vi "Launcher.vi"() -> ()   [LabVIEW 2024]
uses:
  SpeakTurkish/SpeakTurkish.lvclass
  LearnByVisual/LearnByVisual.lvclass
  LearnByReading/LearnByReading.lvclass
  SpeakEnglish/SpeakEnglish.lvclass
  <vilib>/Utility/miscctls.llb/LVRectTypeDef.ctl
  Person/Person.lvclass
panel:
  out "Profile Picture":picture
  in  "Stop":bool
  in  "Person":enum16{"JOHN", "MEHMET", "MARIE"}(ring)
  out "Learning Style":string
  out "Language":string
  out "Name":string
  # "NAME"
  # "SPEAKS"
  # "LEARNS BY"
  # "CHOOSE PERSON"
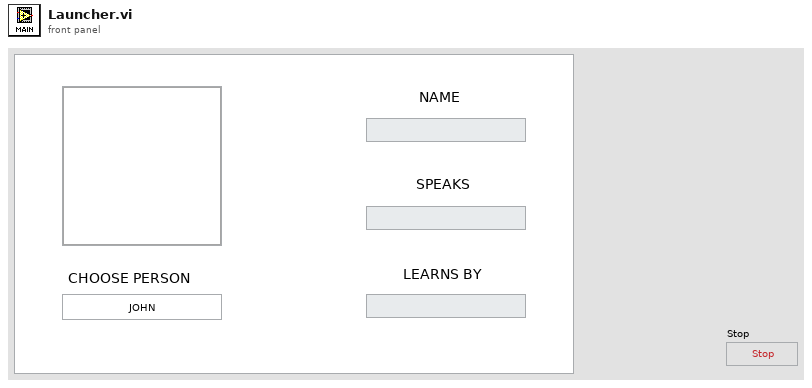
[diagram p1: front panel]
types:
  T1 = typedef "LVRectTypeDef.ctl" = cluster{"Left":i16, "Top":i16, "Right":i16, "Bottom":i16}
  T2 = typedef "LVBoundsTypeDef.ctl" = cluster{"Width":u32, "Height":u32}
  T3 = typedef "imagedata.ctl" = cluster{"image type":i32, "image depth":i32, "image":u8[], "mask":u8[], "colors":u32[], "Rectangle":cluster{"left":i16, "top":i16, "right":i16, "bottom":i16}}
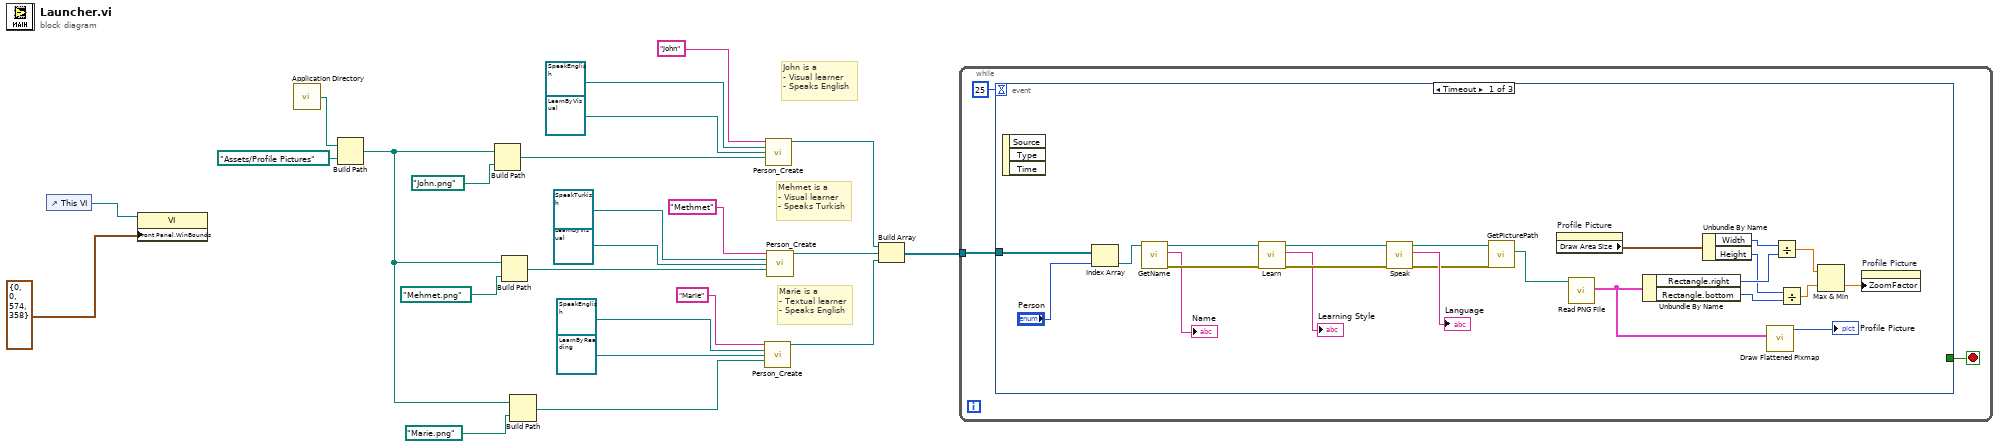
[diagram p0: block diagram]
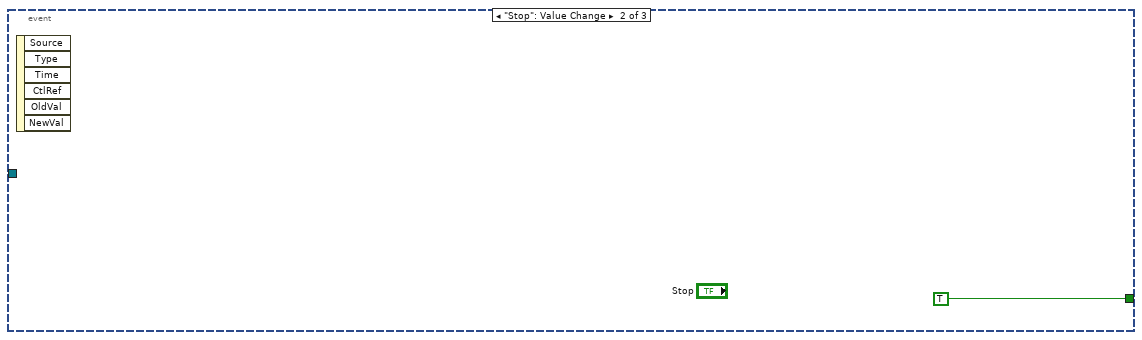
[diagram p2: hidden frame]
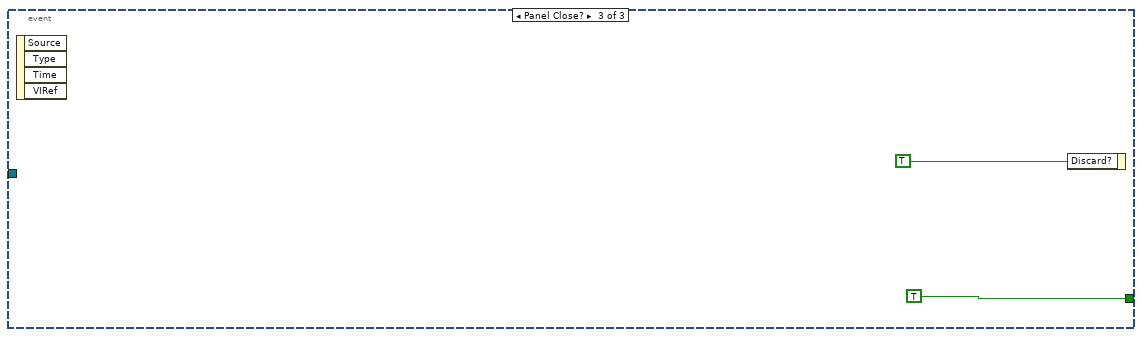
[diagram p3: hidden frame]
diagram:
  # "Marie is a\n- Textual learner\n- Speaks English"
  # "Mehmet is a\n- Visual learner\n- Speaks Turkish"
  # "John is a\n- Visual learner\n- Speaks English"
  n1 = control-ref of="This VI"() -> (w5:refnum<vi>)
  n2 = property class="VI"(reference=w5, "Front Panel.WinBounds"=T1 {"Left"=0, "Top"=0, "Right"=574, "Bottom"=358} ("Front Panel Window:Window Bounds")) -> ()  [unwired: 1 in, 2 out]
  n3 = call <vilib>:"Application Directory.vi"() -> ("Application Directory"=w2:path)
  n4 = Build Path(base path=w2, name or relative path=path "Assets/Profile Pictures") -> (appended path=w3:path)
  n5 = Build Path(base path=w3, name or relative path=path "John.png") -> (appended path=w17:path)
  n6 = Build Path(base path=w3, name or relative path=path "Mehmet.png") -> (appended path=w11:path)
  n7 = Build Path(base path=w3, name or relative path=path "Marie.png") -> (appended path=w6:path)
  n8 = call "Person_Create.vi"("Name"="Marie", "ISpeakBehaviour"=refnum<class "SpeakEnglish.lvclass"> refnum ("SpeakEnglish"), "ILearnBehaviour"=refnum<class "LearnByReading.lvclass"> refnum ("LearnByReading"), "PicturePath"=w6) -> ("reference out"=w22:refnum<class "Person.lvclass">)  [unwired: 10 in, 1 out]
  n9 = call "Person_Create.vi"("Name"="John", "ISpeakBehaviour"=refnum<class "SpeakEnglish.lvclass"> refnum ("SpeakEnglish"), "ILearnBehaviour"=refnum<class "LearnByVisual.lvclass"> refnum ("LearnByVisual"), "PicturePath"=w17) -> ("reference out"=w24:refnum<class "Person.lvclass">)  [unwired: 10 in, 1 out]
  n10 = call "Person_Create.vi"("Name"="Methmet", "ISpeakBehaviour"=refnum<class "SpeakTurkish.lvclass"> refnum ("SpeakTurkish"), "ILearnBehaviour"=refnum<class "LearnByVisual.lvclass"> refnum ("LearnByVisual"), "PicturePath"=w11) -> ("reference out"=w23:refnum<class "Person.lvclass">)  [unwired: 10 in, 1 out]
  n11 = Build Array(w24, w23, w22) -> (w21:refnum<class "Person.lvclass">[])
  n12 = while {
    tunnel: w21 -> [w26]
    stop <- w27 stop-if-true
    n13 = event shown="[0] Timeout" {
      selector: _ -> [_ _ _]
      dyn-events: _ -> [_ _ _]
      timeout: 25 -> [_ _ _]
      tunnel: [_ TRUE TRUE] -> w27
      tunnel: w26 -> [w50 _ _]
      event Timeout {
        n14 = event-data() -> ()  [unwired: 1 in, 3 out]
        n15 = Index Array(array=w50, index="Person") -> (element=w44:refnum<class "Person.lvclass">)
        n16 = call-dynamic "GetName.vi"("reference in"=w44) -> ("Error Out"=w47:errorcluster, "Name"=→"Name":string, "reference out"=w48:refnum<class "Person.lvclass">)  [unwired: 8 in]
        n17 = call-dynamic "Learn.vi"("Error In"=w47, "reference in"=w48) -> ("Error Out"=w45:errorcluster, "Result"=→"Learning Style":string, "reference out"=w46:refnum<class "Person.lvclass">)  [unwired: 7 in]
        n18 = call-dynamic "Speak.vi"("Error In"=w45, "reference in"=w46) -> ("Error Out"=w40:errorcluster, "Result"=→"Language":string, "reference out"=w39:refnum<class "Person.lvclass">)  [unwired: 7 in]
        n19 = call-dynamic "GetPicturePath.vi"("Error In"=w40, "reference in"=w39) -> ("PicturePath"=w37:path)  [unwired: 7 in, 2 out]
        n20 = property on="Profile Picture" class="Pict"() -> ("Draw Area Size"=w38:T2)  [unwired: 2 in, 2 out]
        n21 = call <vilib>:"Read PNG File.vi"("path to PNG file"=w37) -> ("image data"=w30:T3)  [unwired: 8 in, 2 out]
        n22 = Unbundle By Name(w30) -> ("Rectangle.right"=w35:i16, "Rectangle.bottom"=w33:i16)
        n23 = Unbundle By Name(w38) -> ("Width"=w36:u32, "Height"=w34:u32)
        n24 = call <vilib>:"Draw Flattened Pixmap.vi"("image data"=w30) -> ("new picture"=→"Profile Picture":picture)  [unwired: 8 in]
        n25 = Divide(x=w36, y=w35) -> (x/y=w31:dbl)
        n26 = Divide(x=w34, y=w33) -> (x/y=w32:dbl)
        n27 = Max & Min(x=w31, y=w32) -> (min(x,y)=w29:dbl)  [unwired: 1 out]
        n28 = property on="Profile Picture" class="Pict"("ZoomFactor"=w29) -> ()  [unwired: 2 in, 2 out]
      }
      event "Stop": Value Change {
        n29 = event-data() -> ()  [unwired: 1 in, 6 out]
      }
      event Panel Close? {
        n30 = event-data() -> ()  [unwired: 1 in, 4 out]
        n31 = event-data("Discard?"=TRUE) -> ()  [unwired: 1 in, 1 out]
      }
    }
  }
